vi "populate sonde row cluster from sonde data cluster.vi"(7 "Initialize \nInitial Value \nCluster":bool, 8 "error in (no error)":errorcluster, 9 "Sonde Parameters \nInitial Values":T3 {"Salinity Initial" format="%_2f"; "Temp Initial" format="%_2f"; "ORP  Initial" format="%_2f"; "pH Initial" format="%_2f"; "DO Initial" format="%_2f"; "SC Initial" format="%_2f"}, 10 "Sample Sheet Data Row Cluster":T1={"Head\nPressure"=0.0, "Depth"=0.0, "comment string"="", "Sonde Data Cluster"={"Cumulative\nVolume"=100.0, "Specific\nConductance"=2.0, "Dissolved\nOxygen"=3.0, "pH"=4.0, "ORP"=5.0, "Temp"=26.0, "Salinity"=7.0}} {"Sonde Data Cluster"."Salinity" format="%_3g"; "Sonde Data Cluster"."Temp" format="%_2g"; "Sonde Data Cluster"."ORP" format="%_4g"; "Sonde Data Cluster"."pH" format="%_4g"; "Sonde Data Cluster"."Dissolved\nOxygen" format="%_4g"; "Sonde Data Cluster"."Specific\nConductance" format="%_4g"; "Sonde Data Cluster"."Cumulative\nVolume" format="%#_4g"}, 11 "Sonde Parameters \nTolerance Limits":T6 {"Salinity %" format="%_2f%%"; "Temp %" format="%_2f%%"; "ORP %" format="%_2f%%"; "pH %" format="%_2f%%"; "DO %" format="%_2f%%"; "SC %" format="%_2f%%"}) -> (0 "error out":errorcluster, 1 "Cluster":T4 {"Salinity"."%" format="%_2f%%"; "Salinity"."Value" format="%_4g"; "Temperature"."%" format="%_2f%%"; "Temperature"."Value" format="%_4g"; "ORP"."%" format="%_2f%%"; "ORP"."Value" format="%_4g"; "pH"."%" format="%_2f%%"; "pH"."Value" format="%_4g"; "Dissolved Oxygen"."%" format="%_2f%%"; "Dissolved Oxygen"."Value" format="%_4g"; "Sp. Conductance"."%" format="%_2f%%"; "Sp. Conductance"."Value" format="%_4g"; "Cumulative\nVolume" format="%#_4g"}, 6 "Sonde Parameters \nInitial Values Out":T3 {"Salinity Initial" format="%_2f"; "Temp Initial" format="%_2f"; "ORP  Initial" format="%_2f"; "pH Initial" format="%_2f"; "DO Initial" format="%_2f"; "SC Initial" format="%_2f"})   [LabVIEW 2016]
uses:
  activeXtest/activeXtest 2015 Folder/sonde cluster from excel.ctl
  Sonde Value Percent Tol.ctl
  activeXtest/activeXtest 2015 Folder/sample data row cluster.ctl
  activeXtest/activeXtest 2015 Folder/sonde cluster.ctl
panel:
  out "current time":timestamp
  in  "Final":bool
  in  "Input Cluster for % calculation":T4 caption="Cluster" {"Salinity"."%" format="%_2f%%"; "Salinity"."Value" format="%_4g"; "Temperature"."%" format="%_2f%%"; "Temperature"."Value" format="%_4g"; "ORP"."%" format="%_2f%%"; "ORP"."Value" format="%_4g"; "pH"."%" format="%_2f%%"; "pH"."Value" format="%_4g"; "Dissolved Oxygen"."%" format="%_2f%%"; "Dissolved Oxygen"."Value" format="%_4g"; "Sp. Conductance"."%" format="%_2f%%"; "Sp. Conductance"."Value" format="%_4g"; "Cumulative\nVolume" format="%#_4g"}
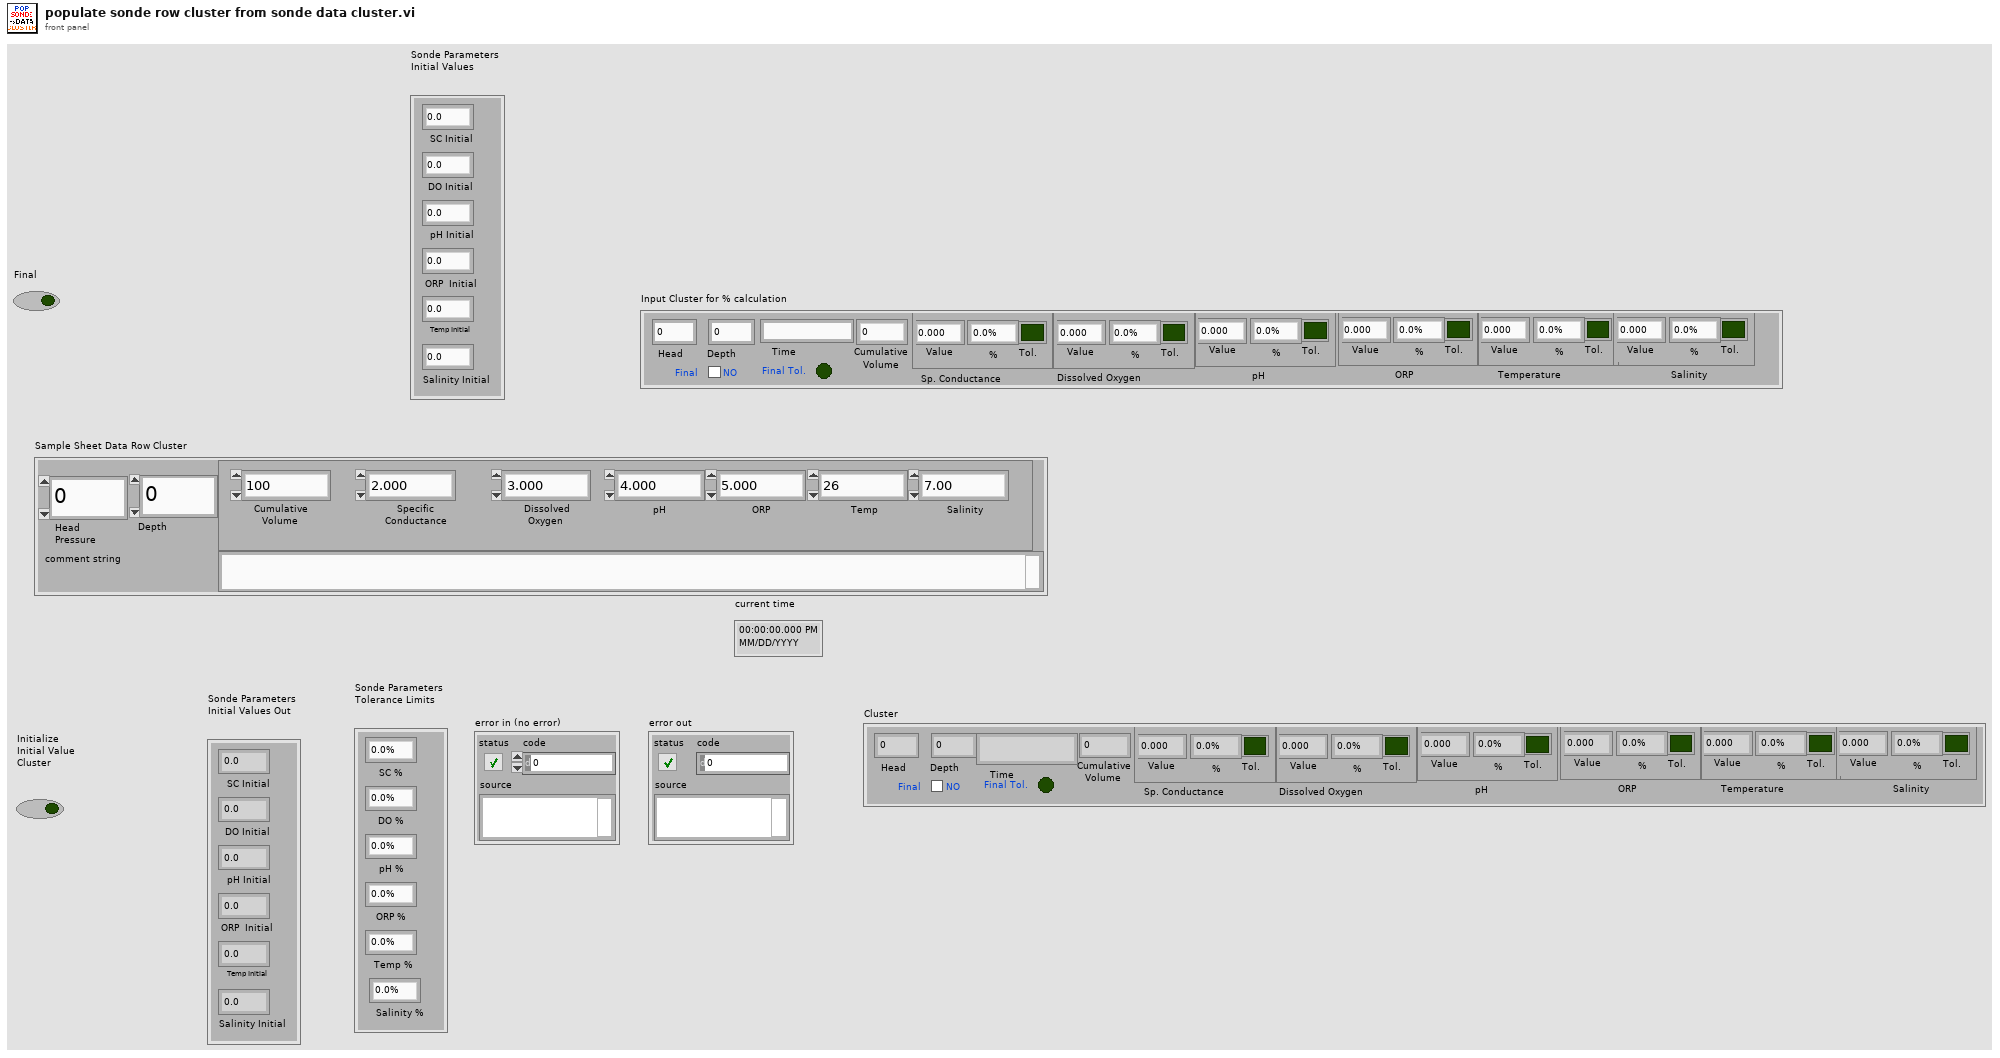
[diagram p1: front panel]
types:
  T1 = typedef "sample data row cluster.ctl" = cluster{"Head\nPressure":dbl, "Depth":dbl, "comment string":string, "Sonde Data Cluster":T2}
  T2 = typedef "sonde cluster.ctl" = cluster{"Cumulative\nVolume":dbl, "Specific\nConductance":dbl, "Dissolved\nOxygen":dbl, "pH":dbl, "ORP":dbl, "Temp":dbl, "Salinity":dbl}
  T3 = cluster{"SC Initial ":dbl, "DO Initial ":dbl, "pH Initial  ":dbl, "ORP  Initial":dbl, "Temp Initial":dbl, "Salinity Initial ":dbl}
  T4 = typedef "sonde cluster from excel.ctl" = cluster{"Head":dbl, "Depth":dbl, "Time":string, "Cumulative\nVolume":dbl, "Sp. Conductance":T5, "Dissolved Oxygen":T5, "pH":T5, "ORP":T5, "Temperature":T5, "Salinity":T5, "Final Tol.":bool, "Final":bool}
  T5 = typedef "Sonde Value Percent Tol.ctl" = cluster{"Value":dbl, "%":dbl, "Tol.":bool}
  T6 = cluster{"SC %":dbl, "DO %":dbl, "pH % ":dbl, "ORP % ":dbl, "Temp % ":dbl, "Salinity %":dbl}
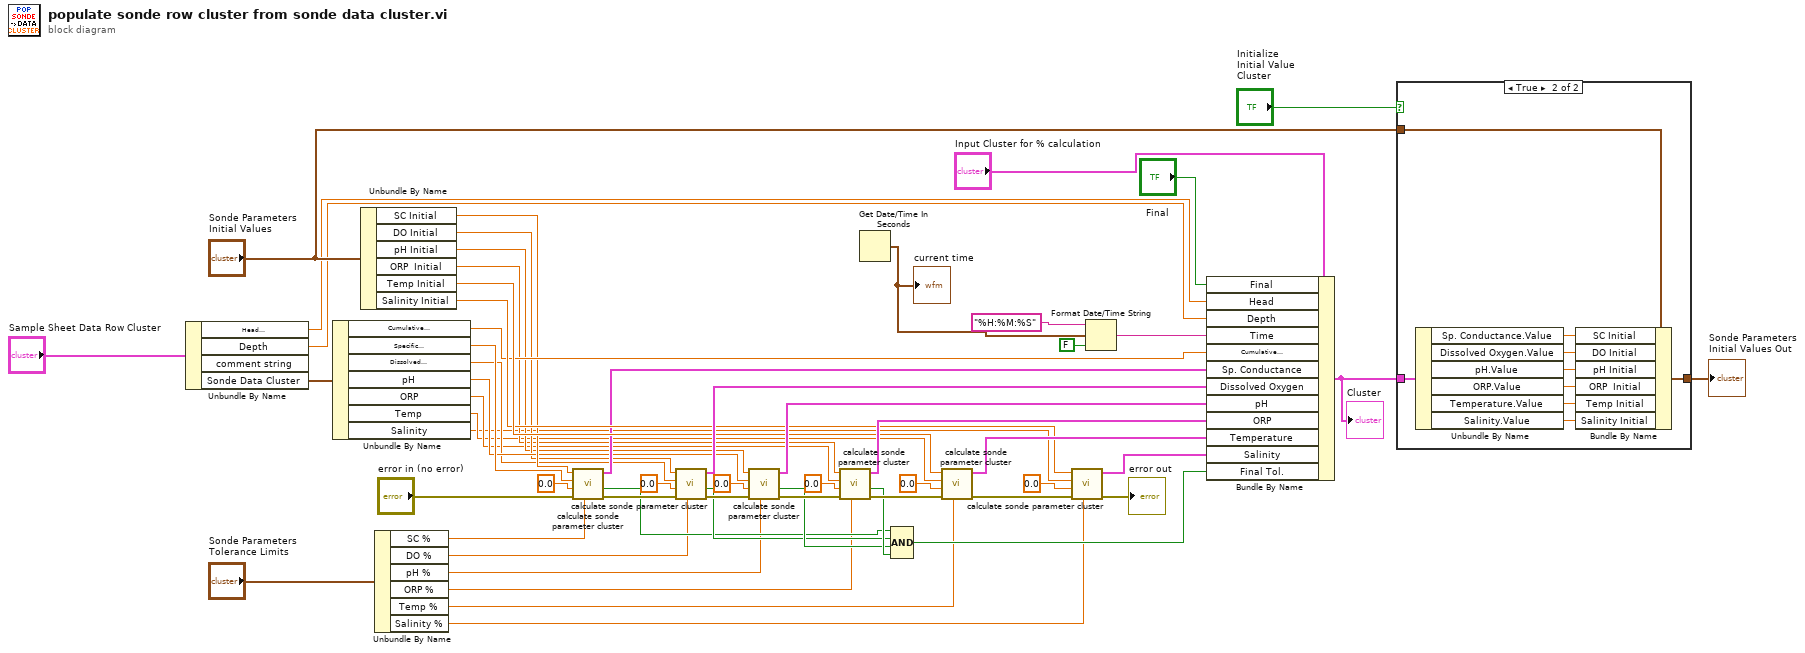
[diagram p0: block diagram]
diagram:
  n1 = Unbundle By Name("Sample Sheet Data Row Cluster") -> ("Head\nPressure"=w30:dbl, "Depth"=w29:dbl, "Sonde Data Cluster"=w28:T2)  [unwired: 1 out]
  n2 = Unbundle By Name(w28) -> ("Cumulative\nVolume"=w27:dbl, "Specific\nConductance"=w22:dbl, "Dissolved\nOxygen"=w16:dbl, "pH"=w18:dbl, "ORP"=w9:dbl, "Temp"=w6:dbl, "Salinity"=w4:dbl)
  n3 = Unbundle By Name("Sonde Parameters \nInitial Values") -> ("SC Initial"=w25:dbl, "DO Initial"=w14:dbl, "pH Initial"=w12:dbl, "ORP  Initial"=w10:dbl, "Temp Initial"=w36:dbl, "Salinity Initial"=w35:dbl)
  n4 = Unbundle By Name("Sonde Parameters \nTolerance Limits") -> ("SC %"=w24:dbl, "DO %"=w13:dbl, "pH %"=w17:dbl, "ORP %"=w8:dbl, "Temp %"=w40:dbl, "Salinity %"=w39:dbl)
  n5 = call "calculate sonde parameter cluster.vi"("tolerance limit"=w24, "error in (no error)"="error in (no error)", "Read % value"=0.0, "Read Value"=w22, "Initial Value"=w25) -> ("error out"=w21:errorcluster, "Tolerance"=w20:bool, "Cluster Out"=w23:T5)  [unwired: 3 in, 1 out]
  n6 = call "calculate sonde parameter cluster.vi"("tolerance limit"=w13, "error in (no error)"=w21, "Read % value"=0.0, "Read Value"=w16, "Initial Value"=w14) -> ("error out"=w57:errorcluster, "Tolerance"=w48:bool, "Cluster Out"=w43:T5)  [unwired: 3 in, 1 out]
  n7 = call "calculate sonde parameter cluster.vi"("tolerance limit"=w17, "error in (no error)"=w57, "Read % value"=0.0, "Read Value"=w18, "Initial Value"=w12) -> ("error out"=w56:errorcluster, "Tolerance"=w49:bool, "Cluster Out"=w44:T5)  [unwired: 3 in, 1 out]
  n8 = call "calculate sonde parameter cluster.vi"("tolerance limit"=w8, "error in (no error)"=w56, "Read % value"=0.0, "Read Value"=w9, "Initial Value"=w10) -> ("error out"=w55:errorcluster, "Tolerance"=w50:bool, "Cluster Out"=w45:T5)  [unwired: 3 in, 1 out]
  n9 = Get Date/Time In Seconds() -> (seconds since 1Jan1904=w1:timestamp)
  "current time" <- w1
  n10 = Compound Arithmetic op=AND(w20, w48, w49, w50) -> (w51:bool)
  n11 = call "calculate sonde parameter cluster.vi"("tolerance limit"=w40, "error in (no error)"=w55, "Read % value"=0.0, "Read Value"=w6, "Initial Value"=w36) -> ("error out"=w54:errorcluster, "Cluster Out"=w46:T5)  [unwired: 3 in, 2 out]
  n12 = call "calculate sonde parameter cluster.vi"("tolerance limit"=w39, "error in (no error)"=w54, "Read % value"=0.0, "Read Value"=w4, "Initial Value"=w35) -> ("error out"=→"error out":errorcluster, "Cluster Out"=w47:T5)  [unwired: 3 in, 2 out]
  n13 = Format Date/Time String(time format string (%c)="%H:%M:%S", seconds (now)=w1, UTC format=FALSE) -> (date/time string=w42:string)
  n14 = Bundle By Name(cluster="Input Cluster for % calculation", "Final"="Final", "Head"=w30, "Depth"=w29, "Time"=w42, "Cumulative\nVolume"=w27, "Sp. Conductance"=w23, "Dissolved Oxygen"=w43, "pH"=w44, "ORP"=w45, "Temperature"=w46, "Salinity"=w47, "Final Tol."=w51) -> (w32:T4)
  "Cluster" <- w32
  n15 = case shown="True" "Initialize \nInitial Value \nCluster" {
    tunnel: "Sonde Parameters \nInitial Values" -> [w59 w68]
    tunnel: [w59 w67] -> w34
    tunnel: w32 -> [_ w66]
    frame False {
    }
    frame True {
      n16 = Unbundle By Name(w66) -> ("Sp. Conductance.Value"=w65:dbl, "Dissolved Oxygen.Value"=w64:dbl, "pH.Value"=w63:dbl, "ORP.Value"=w62:dbl, "Temperature.Value"=w61:dbl, "Salinity.Value"=w60:dbl)
      n17 = Bundle By Name(cluster=w68, "SC Initial"=w65, "DO Initial"=w64, "pH Initial"=w63, "ORP  Initial"=w62, "Temp Initial"=w61, "Salinity Initial"=w60) -> (w67:T3)
    }
  }
  "Sonde Parameters \nInitial Values Out" <- w34
